vi "En-queue RT comms element.vi"(6 "prioritise (F)":bool, 8 "Data":variant, 9 "Message":string, 11 "RT Queues":T1) -> (3 "RT Queues out":T1)   [LabVIEW 2018]
uses:
  Type Defs/Queues cluster.ctl
  ICL-LabVIEW_General/Message Scheduler/message scheduler.lvclass
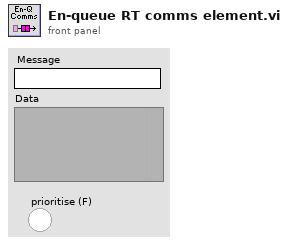
[diagram p1: front panel]
types:
  T1 = typedef "Queues cluster.ctl" = cluster{"RT Message":refnum<queue>, "RT Comms":refnum<queue>, "RT Data":refnum<queue>, "RT FIFO":refnum<queue>, "message scheduler":refnum<class "message scheduler.lvclass">}
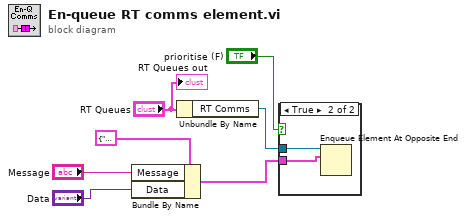
[diagram p0: block diagram]
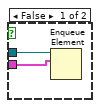
[diagram p2: hidden frame]
diagram:
  n1 = Bundle By Name(cluster=cluster{"Message":string, "Data":variant} {"Message"="", "Data"=variant} ("element"), "Message"="Message", "Data"="Data") -> (w4:cluster{"Message":string, "Data":variant})
  n2 = Unbundle By Name("RT Queues") -> ("RT Comms"=w6:refnum<queue>)
  n3 = case shown="True" "prioritise (F)" {
    tunnel: w6 -> [w9 w11]
    tunnel: w4 -> [w8 w10]
    frame False {
      n4 = Enqueue Element(queue=w9, element=w8) -> ()  [unwired: 2 in, 3 out]
    }
    frame True {
      n5 = Enqueue Element At Opposite End(queue=w11, element=w10) -> ()  [unwired: 2 in, 3 out]
    }
  }
  "RT Queues out" <- "RT Queues"
